vi "Read config file.vi"(8 "error in (no error)":errorcluster, 11 "PS Control Actor in":refnum<class "PS Control Actor.lvclass">) -> (0 "error out":errorcluster, 3 "PS Control Actor out":refnum<class "PS Control Actor.lvclass">)   [LabVIEW 2024, in "PS Control Actor.lvlib" / "PS Control Actor.lvclass"]
uses:
  PS Control Actor.lvclass
  PS Control Actor.lvclass/PS Control Actor.ctl
  <vilib>/Utility/config.llb/Read Key (String).vi
  <vilib>/Utility/config.llb/NI_LVConfig.lvlib
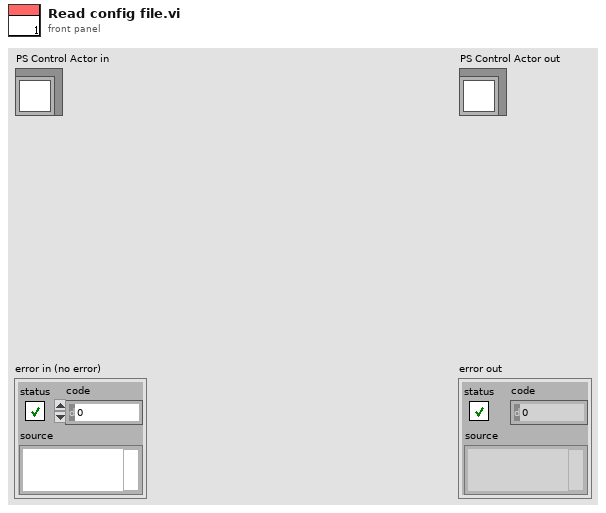
[diagram p1: front panel]
types:
  T1 = typedef "NI_LVConfig.lvlib/Config Data RefNum.ctl" = refnum<k1>
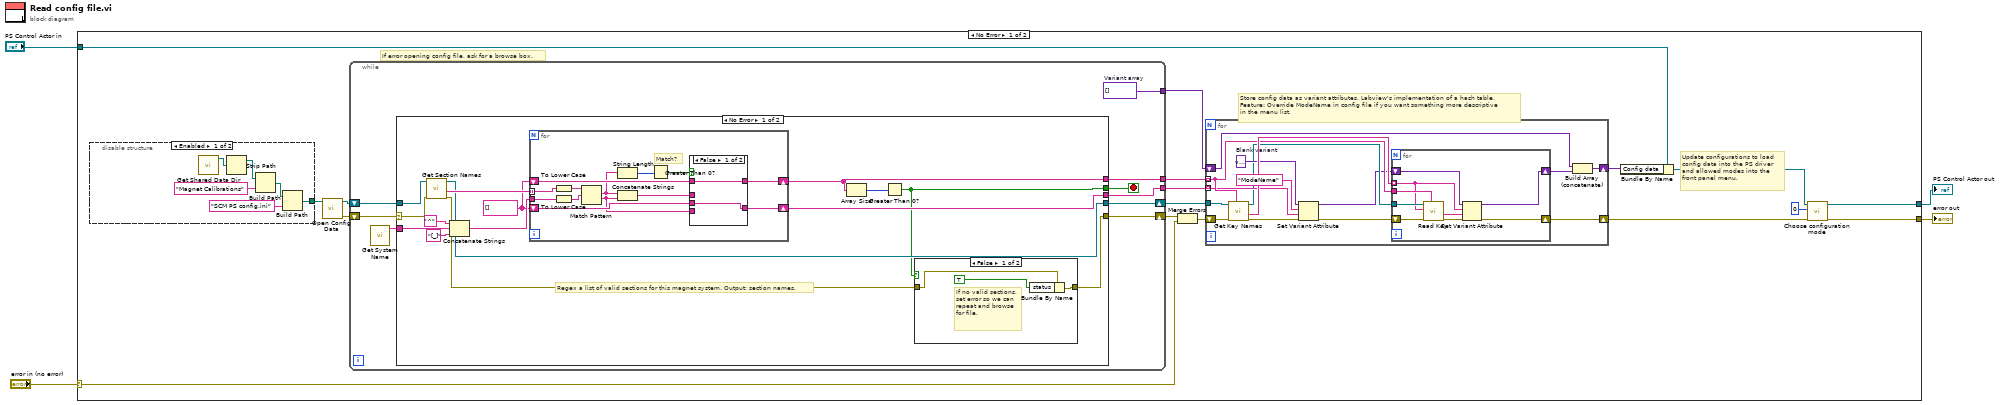
[diagram p0: block diagram]
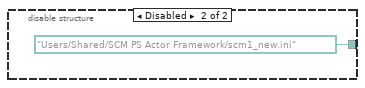
[diagram p2: hidden frame]
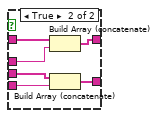
[diagram p4: hidden frame]
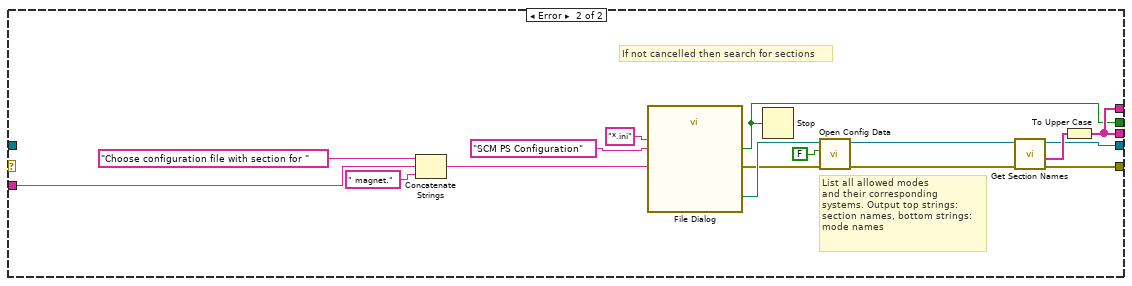
[diagram p5: hidden frame]
diagram:
  n1 = case shown="No Error" "error in (no error)" {
    selector: "error in (no error)" -> [w20 w119]
    tunnel: [w9 w119] -> w3
    tunnel: [w8 w118] -> w1
    tunnel: "PS Control Actor in" -> [w14 w118]
    frame No Error {
      # "Update configurations to load\nconfig data into the PS driver\nand allowed modes into the\nfront panel menu."
      # "Store config data as variant attributes, Labview's implementation of a hash table.\nFeature: Override ModeName in config file if you want something more descriptive\nin the menu list."
      # "If error opening config file, ask for a browse box."
      n2 = disable-structure shown="Enabled" {
        disable-tunnel: [w22 path "/Users/Shared/SCM PS Actor Framework/scm1_new.ini" ("appended path")] -> w6
        frame Enabled {
          n3 = call "Get Shared Data Dir.vi"() -> ("Data Directory Path"=w26:path)  [unwired: 2 in, 1 out]
          n4 = Strip Path(path=w26) -> (stripped path=w25:path)  [unwired: 1 out]
          n5 = Build Path(base path=w25, name or relative path="Magnet Calibrations") -> (appended path=w23:path)
          n6 = Build Path(base path=w23, name or relative path="SCM PS config.ini") -> (appended path=w22:path)
        }
        frame Disabled {
        }
      }
      n7 = call <vilib>:"Open Config Data.vi"("configuration file path"=w6) -> ("error out"=w7:errorcluster, "refnum"=w5:T1)  [unwired: 8 in, 1 out]
      n8 = while {
        tunnel: [w34] -> w18
        tunnel: [w32] -> w16
        tunnel: [w31] -> w15
        shift-right: [w35] -> w19
        shift-left: w7 -> [w37]
        shift-right: [w33] -> w17
        shift-left: w5 -> [w36]
        stop <- w30 stop-if-true
        w31 = variant[] []  # Variant array
        n9 = call "Get System Name.vi"() -> ("System Name"=w29:string)  [unwired: 5 in, 2 out]
        n10 = case shown="No Error" w37 {
          selector: w37 -> [w51 _]
          tunnel: w36 -> [w52 _]
          tunnel: [w39 w85] -> w35
          tunnel: [w42 w83] -> w34
          tunnel: [w46 w84] -> w33
          tunnel: [w44 w83] -> w32
          tunnel: [w41 w78] -> w30
          tunnel: w29 -> [w38 w80]
          frame No Error {
            w45 = string[] []
            # "Regex a list of valid sections for this magnet system. Output: section names."
            n11 = call <vilib>:"Get Section Names.vi"("error in (no error)"=w51, "refnum"=w52) -> ("error out"=w40:errorcluster, "section names"=w50:string[], "refnum out"=w46:T1)  [unwired: 7 in]
            n12 = Concatenate Strings("^", w38, "[_]") -> (w47:string)
            n13 = for {
              tunnel: w50 -> [w60] mode=indexing
              tunnel: w47 -> [w57]
              shift-right: [w67] -> w42
              shift-left: w45 -> [w69]
              shift-right: [w64] -> w44
              shift-left: w45 -> [w66]
              # "Match?"
              n14 = To Lower Case(string=w60) -> (all lower case string=w59:string)
              n15 = To Lower Case(string=w57) -> (all lower case string=w58:string)
              n16 = Match Pattern(string=w59, regular expression=w58) -> (match substring=w62:string, after substring=w65:string)  [unwired: 1 in, 2 out]
              n17 = String Length(string=w62) -> (length=w63:i32)
              n18 = Concatenate Strings(w62, w65) -> (w68:string)
              n19 = Greater Than 0?(x=w63) -> (x > 0?=w61:bool)
              n20 = case shown="False" w61 {
                tunnel: w69 -> [w70 w77]
                tunnel: w68 -> [_ w76]
                tunnel: [w70 w75] -> w67
                tunnel: w66 -> [w71 w74]
                tunnel: w65 -> [_ w73]
                tunnel: [w71 w72] -> w64
                frame False {
                }
                frame True {
                  n21 = Build Array (concatenate)(w77, w76) -> (w75:string[])
                  n22 = Build Array (concatenate)(w74, w73) -> (w72:string[])
                }
              }
            }
            n23 = Array Size(array=w42) -> (size(s)=w43:i32)
            n24 = Greater Than 0?(x=w43) -> (x > 0?=w41:bool)
            n25 = case shown="False" w41 {
              tunnel: w40 -> [w54 w56]
              tunnel: [w55 w56] -> w39
              frame False {
                # "If no valid sections, set error so we can repeat and browse for file."
                n26 = Bundle By Name(cluster=w54, "status"=TRUE) -> (w55:errorcluster)
              }
              frame True {
              }
            }
          }
          frame Error {
            # "If not cancelled then search for sections"
            # "List all allowed modes\nand their corresponding\nsystems. Output top strings: \nsection names, bottom strings:\nmode names"
            n27 = Concatenate Strings("Choose configuration file with section for " ("prompt"), w80, " magnet." ("string")) -> (w81:string)
            n28 = call "File Dialog"("prompt"=w81, "pattern (all files)"="*.ini", "pattern label"="SCM PS Configuration") -> ("selected path"=w89:path, "cancelled"=w78:bool, "error out"=w88:errorcluster)  [unwired: 9 in, 1 out]
            n29 = Stop(stop? (T)=w78) -> ()
            n30 = call <vilib>:"Open Config Data.vi"("error in (no error)"=w88, "create file if necessary (T)"=FALSE ("create file if necessary? (T)"), "configuration file path"=w89) -> ("error out"=w82:errorcluster, "refnum"=w87:T1)  [unwired: 6 in, 1 out]
            n31 = call <vilib>:"Get Section Names.vi"("error in (no error)"=w82, "refnum"=w87) -> ("error out"=w85:errorcluster, "section names"=w86:string[], "refnum out"=w84:T1)  [unwired: 7 in]
            n32 = To Upper Case(1:w86) -> (0:w83:string[])
          }
        }
      }
      n33 = Merge Errors(w19, w20) -> (w21:errorcluster)
      n34 = for {
        shift-right: [w102] -> w10
        shift-left: w21 -> [w108]
        tunnel: w18 -> [w103] mode=indexing
        tunnel: w17 -> [w107]
        tunnel: w16 -> [w98] mode=indexing
        shift-right: [w105] -> w13
        shift-left: w15 -> [w106]
        w99 = variant  # Blank variant
        n35 = call <vilib>:"Get Key Names.vi"("section"=w103, "error in (no error)"=w108, "refnum"=w107) -> ("error out"=w97:errorcluster, "key names"=w104:string[], "refnum out"=w96:T1)  [unwired: 5 in, 1 out]
        n36 = Set Variant Attribute(Variant=w99, name="ModeName", value=w98, error in=w97) -> (Variant out=w94:variant, error out=w95:errorcluster)  [unwired: 1 out]
        n37 = for {
          tunnel: w104 -> [w111] mode=indexing
          tunnel: w103 -> [w117]
          tunnel: w96 -> [w116]
          shift-right: [w113] -> w102
          shift-left: w95 -> [w115]
          shift-right: [w109] -> w101
          shift-left: w94 -> [w110]
          n38 = call-poly <vilib>:"Read Key.vi"("section"=w117, "error in (no error)"=w115, "key"=w111, "refnum"=w116) -> ("error out"=w114:errorcluster, "value"=w112:string)  [unwired: 4 in, 2 out]
          n39 = Set Variant Attribute(Variant=w110, name=w111, value=w112, error in=w114) -> (Variant out=w109:variant, error out=w113:errorcluster)  [unwired: 1 out]
        }
        n40 = Build Array (concatenate)(w106, w101) -> (w105:variant[])
      }
      n41 = Bundle By Name(cluster=w14, "Config data"=w13) -> (w12:refnum<class "PS Control Actor.lvclass">)
      n42 = call "Choose configuration mode.vi"("error in (no error)"=w10, "Choose configuration mode"=u16 0, "PS Control Actor in"=w12) -> ("error out"=w9:errorcluster, "PS Control Actor out"=w8:refnum<class "PS Control Actor.lvclass">)  [unwired: 7 in]
    }
    frame Error {
    }
  }
  "error out" <- w3
  "PS Control Actor out" <- w1
